vi "实验3-4.vi"() -> ()   [LabVIEW 2018]
panel:
  in  "停止":bool
  out "位置":cluster{"宽度":dbl, "高度":dbl}
  in  "位置":cluster{"左":dbl, "上":dbl}
  in  "̬焦点状态":bool
  in  "闪烁2":bool
  in  "禁用":u16
  in  "可见控制":bool
  in  "数值":dbl
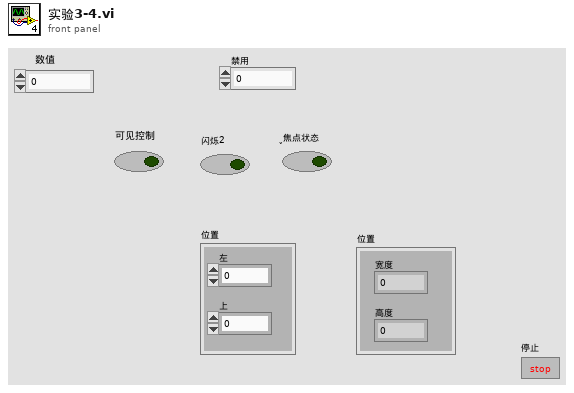
[diagram p1: front panel]
types:
  T1 = typedef "LVBoundsTypeDef.ctl" = cluster{"Width":u32, "Height":u32}
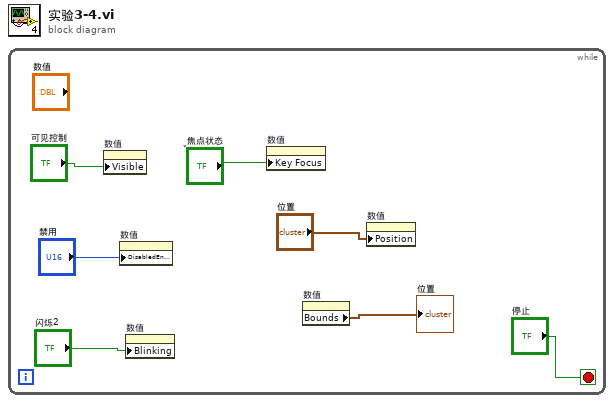
[diagram p0: block diagram]
diagram:
  n1 = while {
    stop <- "停止" stop-if-true
    n2 = property on="数值" class="DigNum (strict)"("Visible"="可见控制") -> ()  [unwired: 2 in, 2 out]
    n3 = property on="数值" class="DigNum (strict)"("DisabledEnum"="禁用") -> ()  [unwired: 2 in, 2 out]
    n4 = property on="数值" class="DigNum (strict)"("Blinking"="闪烁2") -> ()  [unwired: 2 in, 2 out]
    n5 = property on="数值" class="DigNum (strict)"("Key Focus"="̬焦点状态") -> ()  [unwired: 2 in, 2 out]
    n6 = property on="数值" class="DigNum (strict)"() -> ("Bounds"=→"位置":T1)  [unwired: 2 in, 2 out]
    n7 = property on="数值" class="DigNum (strict)"("Position"="位置") -> ()  [unwired: 2 in, 2 out]
  }
